vi "SettingPanelOtherDivice.vi"(11 "OtherDivice_In":refnum<vi>) -> (3 "OtherDivice_Out":refnum<vi>)   [LabVIEW 2013]
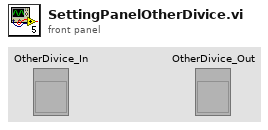
[diagram p1: front panel]
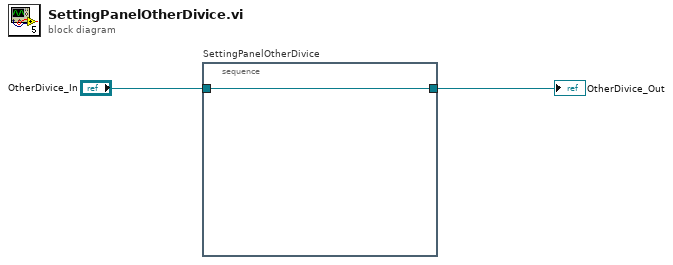
[diagram p0: block diagram]
diagram:
  n1 = stacked-sequence "SettingPanelOtherDivice" {
    tunnel: "OtherDivice_In" -> [w3]
    tunnel: [w3] -> w2
    frame #0 {
    }
  }
  "OtherDivice_Out" <- w2
